vi "MainT3.vi"() -> ()   [LabVIEW 2019]
uses:
  <instrlib>/niDMM/nidmm.llb/niDMM Function.ctl
  <instrlib>/niDMM/nidmm.llb/niDMM Resolution in Digits.ctl
panel:
  in  "stop":bool
  in  "Self-Calibrate Multimeter at the beginning?":bool
  in  "Tab Control":T1(tab)
  out "Waveform Chart 2":cluster{dbl, dbl, dbl}(graph)
  in  "Recieve Data":bool
  in  "VISA resource name":refnum<visa-resource-name>="COM3"
  in  "termination char\n(0xA = '\\n' = LF)":u8=13 format="%.0x"
  out "Waveform Chart 4":T2(graph)
  in  "resistance configuration":i32(ring)=2 items=["2-Wire"=2, "3-Wire"=3, "4-Wire"=4]
  in  "Range (Volts)":dbl=10.0 format="%.2p"
  in  "physical channels":tag="PXI1Slot2/ai3"
  out "Thermometer":dbl(slide) scale=0.0..100.0
  in  "selection":i32
  out "Waveform Chart 3":dbl(graph)
  out "Over Range?":bool
  in  "Instrument Descriptor":refnum<k15>="PXI1Slot4"
  in  "Function":T3
  in  "Resolution in Digits":T4=5.5 items=["3 1/2"=3.5, "4 1/2"=4.5, "5 1/2"=5.5, "6 1/2"=6.5, "7 1/2"=7.5]
  out "Measurement (Volts)":dbl format="%_5p"
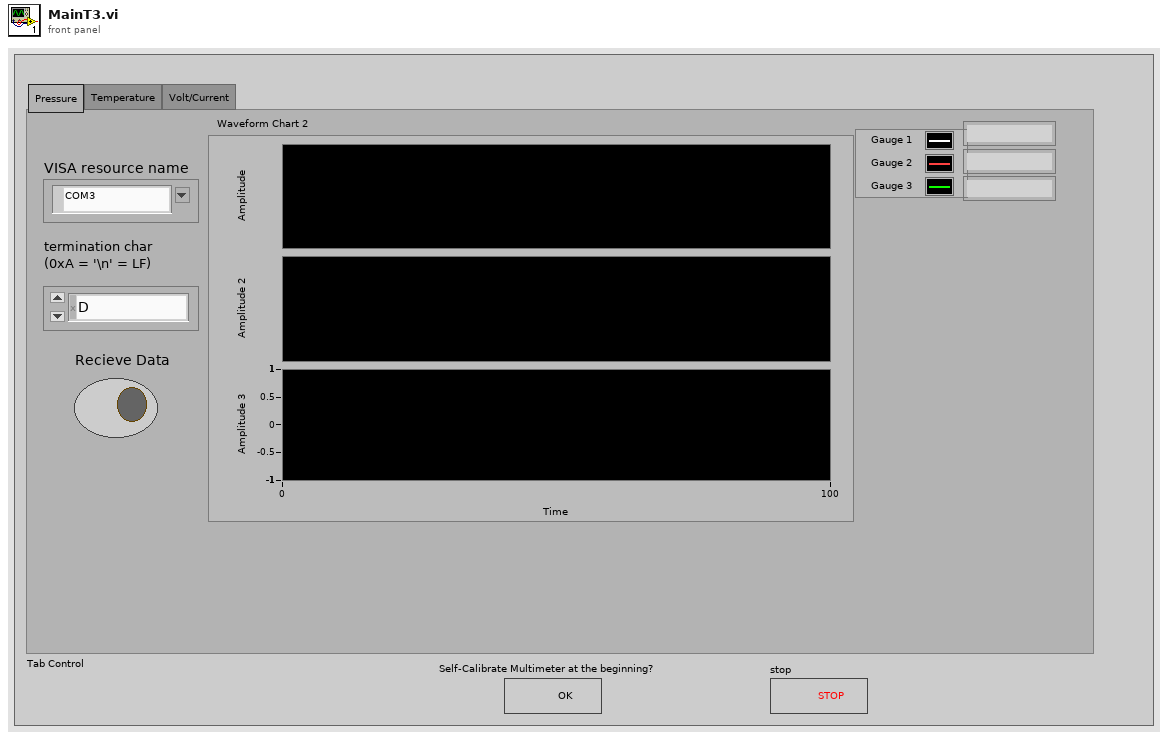
[diagram p1: front panel]
types:
  T1 = enum32{"Pressure", "Temperature", "Volt/Current"}
  T2 = cluster{"data[0]":dbl, "data[1]":dbl, "data[2]":dbl, "data[3]":dbl, "data[4]":dbl, "data[5]":dbl, "data[6]":dbl, "data[7]":dbl, "data[8]":dbl}
  T3 = typedef "niDMM Function.ctl" = enum16{"DC Volts", "AC Volts", "DC Current", "AC Current", "2-wire Resistance", "4-wire Resistance", "Diode", "Frequency", "Period", "AC Volts DC Coupled", "Capacitance", "Inductance", "Temperature"}
  T4 = typedef "niDMM Resolution in Digits.ctl" = dbl
  T5 = enum16{"open", "replace", "create", "open or create", "replace or create", "replace or create with confirmation"}
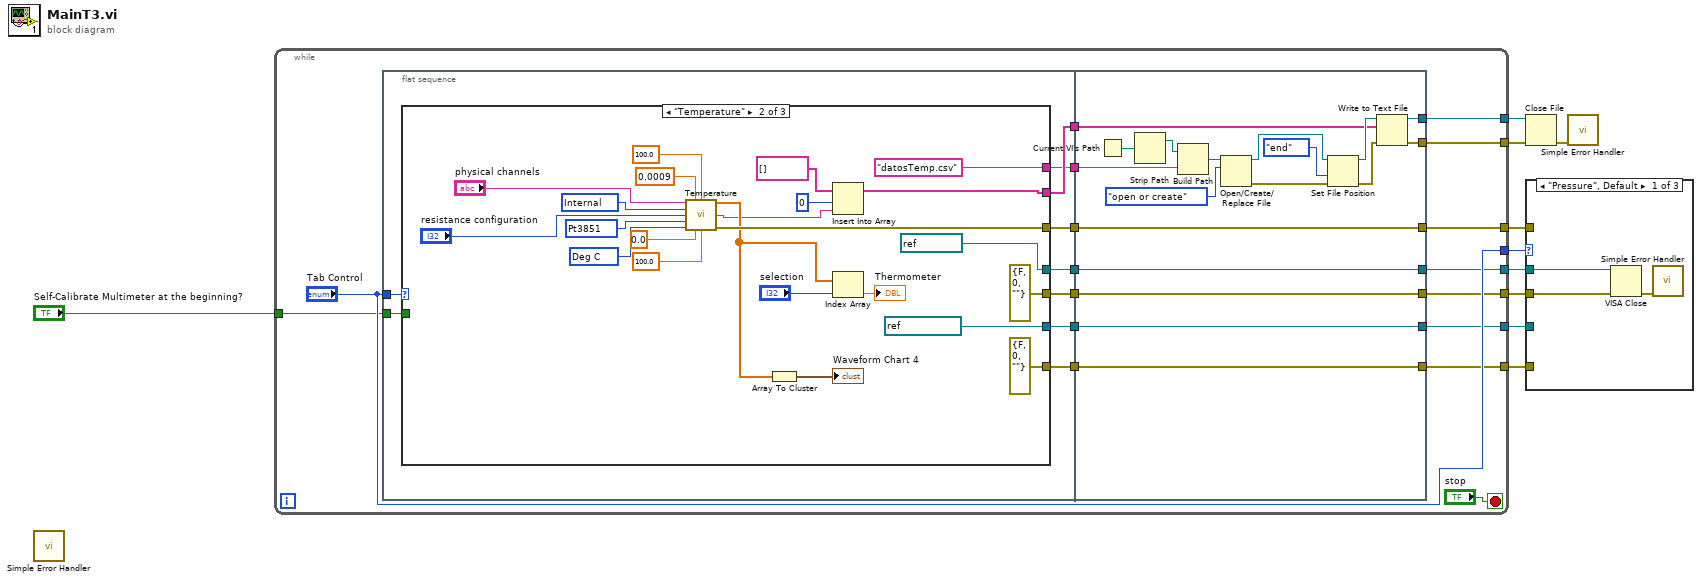
[diagram p0: block diagram]
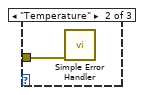
[diagram p2: hidden frame]
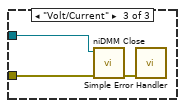
[diagram p3: hidden frame]
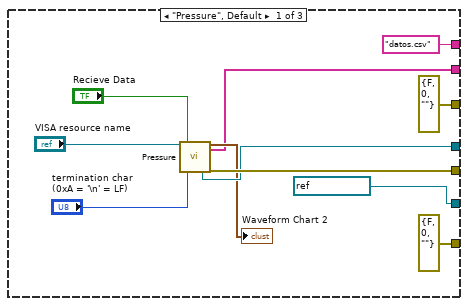
[diagram p4: hidden frame]
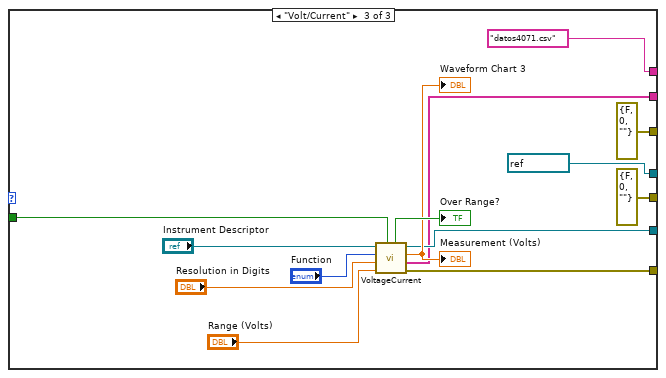
[diagram p5: hidden frame]
diagram:
  n1 = call <vilib>:"Simple Error Handler.vi"() -> ()  [unwired: 5 in, 5 out]
  n2 = while {
    tunnel: "Self-Calibrate Multimeter at the beginning?" -> [w25]
    tunnel: [w24] -> w8
    tunnel: [w23] -> w7
    tunnel: [w22] -> w6
    tunnel: [w21] -> w5
    tunnel: [w20] -> w4
    tunnel: ["Tab Control"] -> w9
    tunnel: [w11] -> w2
    tunnel: [w12] -> w1
    stop <- "stop" stop-if-true
    n3 = flat-sequence {
      tunnel: "Tab Control" -> [w36]
      tunnel: w25 -> [w35]
      tunnel: [w34] -> w19
      tunnel: [w33] -> w18
      tunnel: [w32] -> w17
      tunnel: [w31] -> w16
      tunnel: [w30] -> w15
      tunnel: [w29] -> w14
      tunnel: [w28] -> w13
      tunnel: [w98] -> w20
      tunnel: [w99] -> w21
      tunnel: [w100] -> w22
      tunnel: [w101] -> w23
      tunnel: [w102] -> w24
      tunnel: w19 -> [w102]
      tunnel: w18 -> [w101]
      tunnel: w17 -> [w100]
      tunnel: w16 -> [w99]
      tunnel: w15 -> [w98]
      tunnel: w14 -> [w89]
      tunnel: w13 -> [w90]
      tunnel: [w86] -> w12
      tunnel: [w85] -> w11
      frame #0 {
        n4 = case shown="\"Temperature\"" w36 {
          tunnel: w35 -> [_ _ w79]
          tunnel: [w44 errorcluster {"status"=FALSE, "code"=0, "source"=""} ("error out") errorcluster {"status"=FALSE, "code"=0, "source"=""} ("error out")] -> w34
          tunnel: [w43 refnum<visa-resource-name> "COM3" ("VISA resource name out") refnum<visa-resource-name> "COM3" ("VISA resource name out")] -> w33
          tunnel: [errorcluster {"status"=FALSE, "code"=0, "source"=""} ("error out") w61 errorcluster {"status"=FALSE, "code"=0, "source"=""} ("error out")] -> w32
          tunnel: [errorcluster {"status"=FALSE, "code"=0, "source"=""} ("error out") errorcluster {"status"=FALSE, "code"=0, "source"=""} ("error out") w76] -> w31
          tunnel: [refnum<k15> "PXI1Slot4" ("instrument handle out") refnum<k15> "PXI1Slot4" ("instrument handle out") w75] -> w30
          tunnel: [w41 w49 w72] -> w29
          tunnel: ["datos.csv" ("name or relative path") "datosTemp.csv" ("name or relative path") "datos4071.csv" ("name or relative path")] -> w28
          frame "Pressure", Default {
            n5 = call "Pressure.vi"("VISA resource name"="VISA resource name", "Recieve Data"="Recieve Data", "termination char\n(0xA = '\\n' = LF)"="termination char\n(0xA = '\\n' = LF)") -> ("VISA resource name out"=w43:refnum<visa-resource-name>, "output cluster"=→"Waveform Chart 2":cluster{dbl, dbl, dbl}, "output array"=w41:string[], "error out"=w44:errorcluster)  [unwired: 10 in, 3 out]
          }
          frame "Temperature" {
            w64 = 10143 items=["Deg C"=10143, "Deg F"=10144, "Kelvins"=10325, "Deg R"=10145, "From Custom Scale"=10065] ("units")
            w65 = 10071 items=["Pt3750"=12481, "Pt3851"=10071, "Pt3911"=12482, "Pt3916"=10069, "Pt3920"=10053, "Pt3928"=12483, "Custom"=10137] ("rtd type")
            w66 = 10200 items=["Internal"=10200, "External"=10167, "None"=10230] ("current excitation source")
            n6 = call "Temperature.vi"("physical channels"="physical channels", "current excitation value"=0.0009, "r0"=100.0, "current excitation source"=w66, "resistance configuration"="resistance configuration", "rtd type"=w65, "units"=w64, "minimum value"=0.0, "maximum value"=100.0) -> ("data"=w58:dbl[], "spreadsheet string"=w48:string, "error out"=w61:errorcluster)  [unwired: 4 in]
            n7 = Array To Cluster(array=w58) -> (cluster=→"Waveform Chart 4":T2)
            n8 = Insert Into Array(array=string[] [], index=0, new element=w48) -> (w49:string[])
            n9 = Index Array(array=w58, index="selection") -> (element=→"Thermometer":dbl)
          }
          frame "Volt/Current" {
            n10 = call "VoltageCurrent.vi"("Self-Calibrate at the beginning?"=w79, "Range (Volts)"="Range (Volts)", "Resolution in Digits"="Resolution in Digits", "Function"="Function", "Instrument Descriptor"="Instrument Descriptor") -> ("error out"=w76:errorcluster, "output array"=w72:string[], "Measurement (Volts)"=→"Waveform Chart 3" →"Measurement (Volts)":dbl, "instrument handle out"=w75:refnum<k15>, "Over Range?"=→"Over Range?":bool)  [unwired: 2 in]
          }
        }
      }
      frame #1 {
        n11 = Current VI's Path() -> (path=w97:path)
        n12 = Strip Path(path=w97) -> (stripped path=w96:path)  [unwired: 1 out]
        n13 = Build Path(base path=w96, name or relative path=w90) -> (appended path=w94:path)
        n14 = Open/Create/Replace File(file path (use dialog)=w94, operation (0:open)=T5."open or create") -> (refnum out=w93:refnum<file>, error out=w91:errorcluster)  [unwired: 4 in, 1 out]
        n15 = Set File Position(refnum=w93, from (0:start)=enum16{"start", "end", "current"}."end", error in=w91) -> (refnum out=w95:refnum<file>, error out=w92:errorcluster)  [unwired: 1 in]
        n16 = Write to Text File(file (use dialog)=w95, text=w89, error in=w92) -> (refnum out=w85:refnum<file>, error out=w86:errorcluster)  [unwired: 1 in, 1 out]
      }
    }
  }
  n17 = Close File(refnum=w2, error in=w1) -> (error out=w3:errorcluster)  [unwired: 1 out]
  n18 = case shown="\"Pressure\", Default" w9 {
    tunnel: w8 -> [w104 _ _]
    tunnel: w7 -> [w103 _ _]
    tunnel: w6 -> [_ w106 _]
    tunnel: w5 -> [_ _ w108]
    tunnel: w4 -> [_ _ w107]
    frame "Pressure", Default {
      n19 = VISA Close(VISA resource name=w103, error in (no error)=w104) -> (error out=w105:errorcluster)
      n20 = call <vilib>:"Simple Error Handler.vi"("error in (no error)"=w105) -> ()  [unwired: 4 in, 5 out]
    }
    frame "Temperature" {
      n21 = call <vilib>:"Simple Error Handler.vi"("error in (no error)"=w106) -> ()  [unwired: 4 in, 5 out]
    }
    frame "Volt/Current" {
      n22 = call <instrlib>:"niDMM Close.vi"("error in (no error)"=w108, "instrument handle"=w107) -> ("error out"=w109:errorcluster)  [unwired: 9 in]
      n23 = call <vilib>:"Simple Error Handler.vi"("error in (no error)"=w109) -> ()  [unwired: 4 in, 5 out]
    }
  }
  n24 = call <vilib>:"Simple Error Handler.vi"("error in (no error)"=w3) -> ()  [unwired: 1 in, 8 out]
